vi "Path.vi"(8 "error in (no error)":errorcluster, 10 "pathname":string, 11 "Master in":refnum<class "Master.lvclass">) -> (0 "error out":errorcluster, 3 "Master out":refnum<class "Master.lvclass">)   [LabVIEW 2014, in "Master.lvclass"]
uses:
  Master/Master.lvclass
  Master/Master.lvclass/Master.ctl
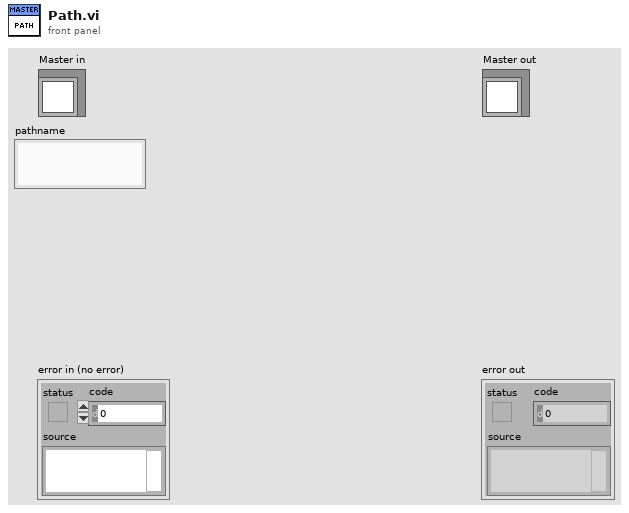
[diagram p1: front panel]
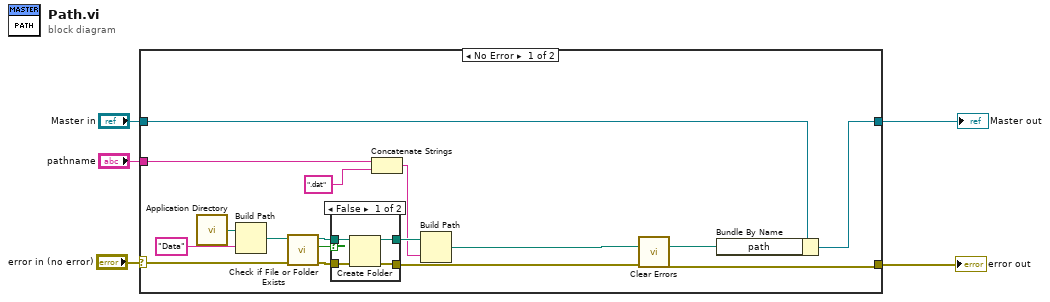
[diagram p0: block diagram]
diagram:
  n1 = case shown="No Error" "error in (no error)" {
    selector: "error in (no error)" -> [w18 w29]
    tunnel: [w6 w29] -> w4
    tunnel: [w10 w28] -> w2
    tunnel: "Master in" -> [w8 w28]
    tunnel: "pathname" -> [w11 _]
    frame No Error {
      n2 = call <vilib>:"Application Directory.vi"() -> ("Application Directory"=w21:path)
      n3 = Build Path(base path=w21, name or relative path="Data") -> (appended path=w19:path)
      n4 = call <vilib>:"Check if File or Folder Exists.vi"("error in (no error)"=w18, "path"=w19) -> ("error out"=w15:errorcluster, "file or folder exists?"=w17:bool, "dup path"=w16:path)  [unwired: 7 in]
      n5 = case shown="False" w17 {
        tunnel: w16 -> [w25 w27]
        tunnel: w15 -> [w24 w26]
        tunnel: [w23 w27] -> w14
        tunnel: [w22 w26] -> w7
        frame False {
          n6 = Create Folder(path (use dialog)=w25, error in=w24) -> (created path=w23:path, error out=w22:errorcluster)  [unwired: 1 in, 1 out]
        }
        frame True {
        }
      }
      n7 = Concatenate Strings(w11, ".dat" ("string")) -> (w13:string)
      n8 = Build Path(base path=w14, name or relative path=w13) -> (appended path=w9:path)
      n9 = call <vilib>:"Clear Errors.vi"("error in (no error)"=w7) -> ("error out"=w6:errorcluster)  [unwired: 5 in, 1 out]
      n10 = Bundle By Name(cluster=w8, "path"=w9) -> (w10:refnum<class "Master.lvclass">)
    }
    frame Error {
    }
  }
  "error out" <- w4
  "Master out" <- w2
